vi "GenerateTestAllTask.vi"() -> (3 "Task Out":refnum<k21>)   [LabVIEW 2013]
uses:
  <vilib>/DAQmx/create/channels.llb/DAQmx Create Channel (AI-Voltage-Basic).vi
  <vilib>/DAQmx/create/channels.llb/DAQmx Create Channel (AI-Strain-Strain Gage).vi
  <vilib>/DAQmx/create/channels.llb/DAQmx Create Channel (AI-Position-LVDT).vi
  <vilib>/DAQmx/create/channels.llb/DAQmx Create Channel (AI-Position-RVDT).vi
  Instance           1 27Saved   GenerateTestAllTask .vi
  <resource>/objmgr/daqmx.rc
  Popups/Progress Bar Actions.ctl
  Data Access Objects/Channel Paths/Channel Path List Actions.ctl
panel:
  out "error out":errorcluster
  in  "error in (no error)":errorcluster
  out "Name":string
  out "AI.MeasType":i32(ring)=10300 items=["Voltage"=10322, "Current"=10134, "More:Voltage:Custom with Excitation"=10323, "Frequency"=10181, "Resistance"=10278, "Temperature:Thermocouple"=10303, "Temperature:Thermistor"=10302, "Temperature:RTD"=10301, "Temperature:Built-in Sensor"=10311, "Strain Gage"=10300, "Position:LVDT"=10352, "Position:RVDT"=10353, "Accelerometer"=10356, "Sound Pressure:Microphone"=10354, "TEDS Sensor"=12531]
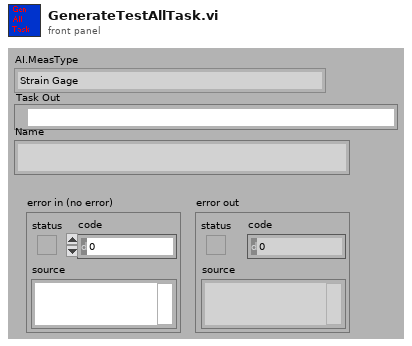
[diagram p1: front panel]
types:
  T1 = typedef "Channel Path List Actions.ctl" = enum16{"Set List", "Get Cont List", "Get Step List", "Get OM List", "Get All List", "Get Exc List", "Get Base List", "Sort List"}
  T2 = typedef "Progress Bar Actions.ctl" = enum16{"Get", "Set", "Exit", "Init"}
  T3 = cluster{"gage factor":dbl, "nominal gage resistance":dbl, "poisson ratio":dbl}
  T4 = cluster{"strain configuration":i32, "lead wire resistance":dbl, "initial bridge voltage":dbl, "voltage excitation source":i32, "voltage excitation value":dbl}
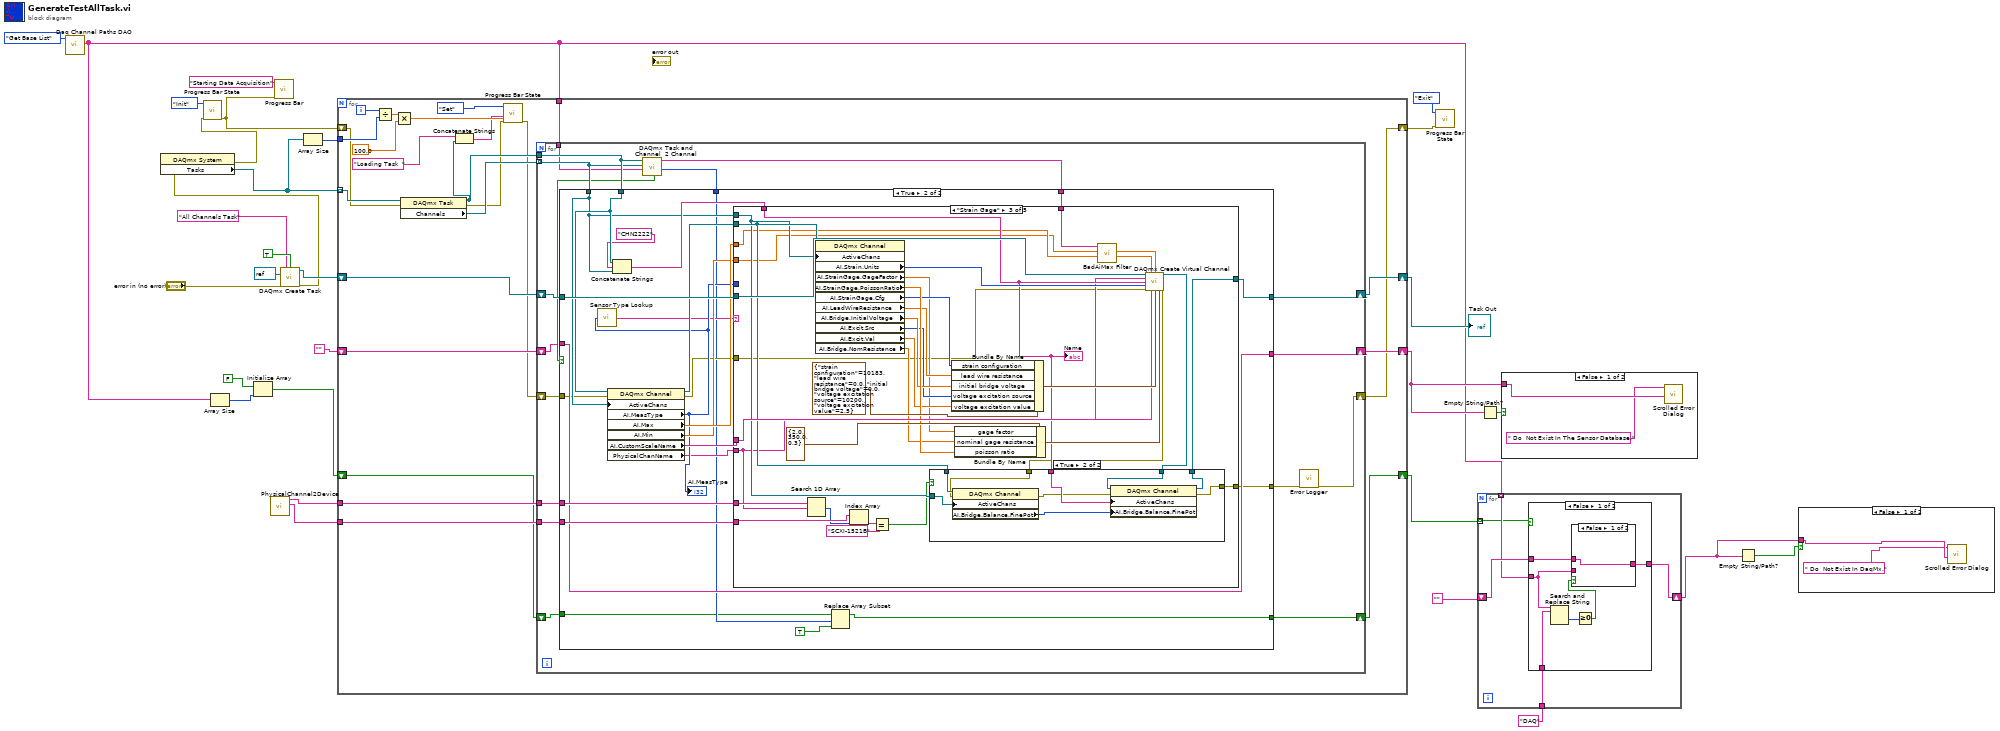
[diagram p0: block diagram]
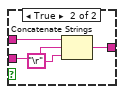
[diagram p3: hidden frame]
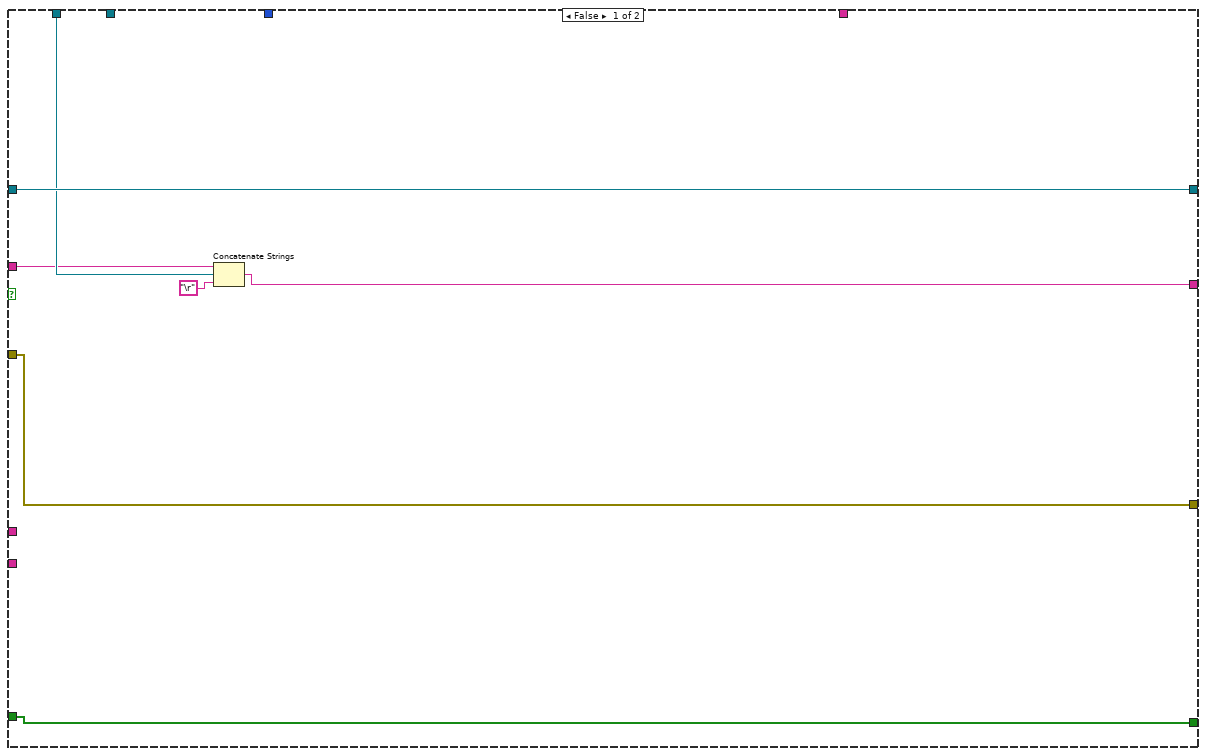
[diagram p6: hidden frame]
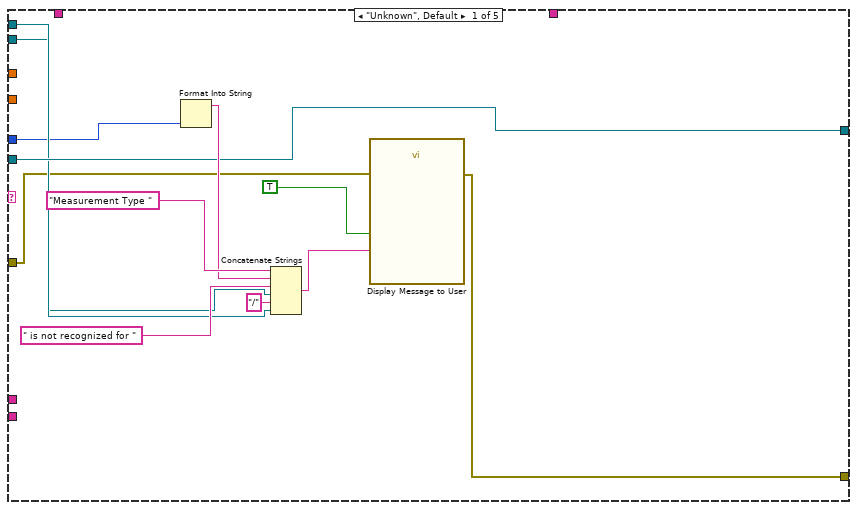
[diagram p7: hidden frame]
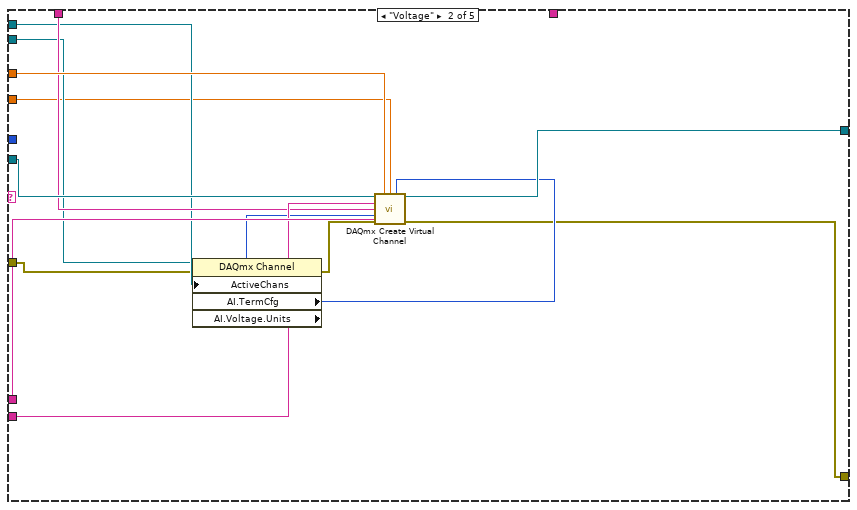
[diagram p8: hidden frame]
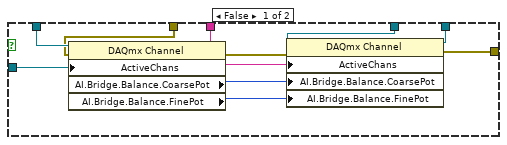
[diagram p9: hidden frame]
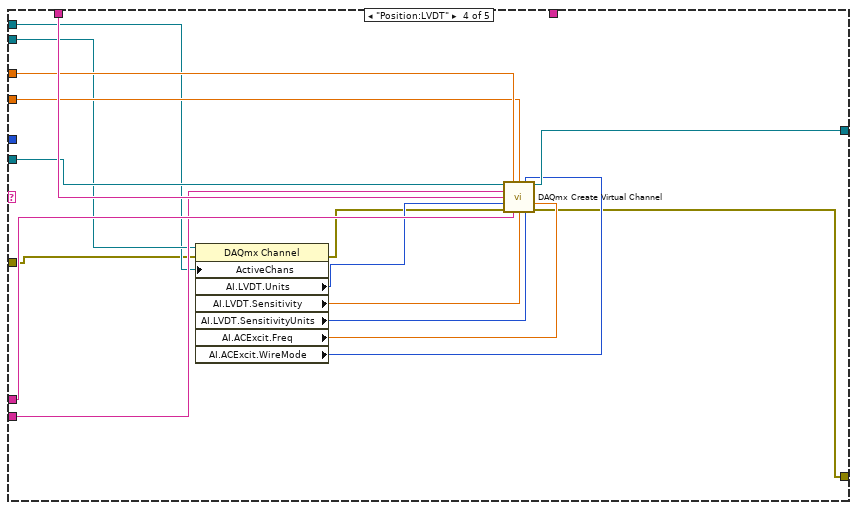
[diagram p10: hidden frame]
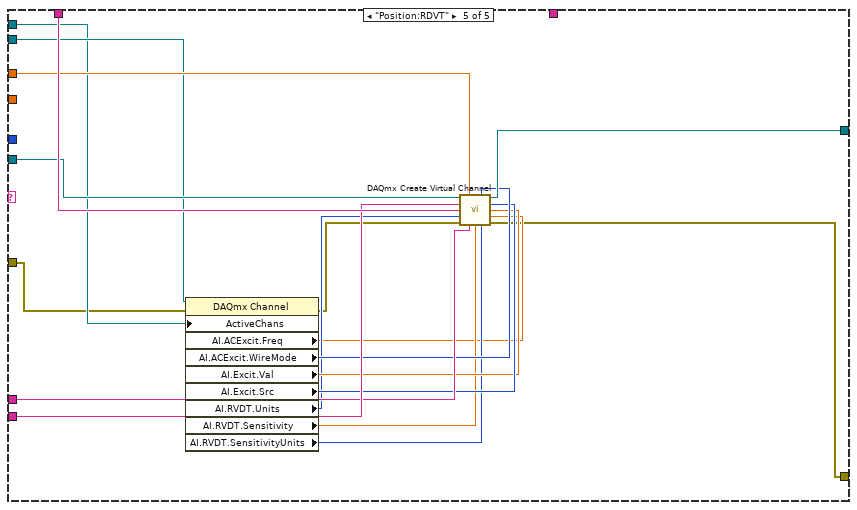
[diagram p11: hidden frame]
diagram:
  n1 = call "Daq Channel Paths DAO.vi"("Actions"=Channel_Path_List_Actions."Get Base List") -> ("Channel Path List Out"=w7:string[])  [unwired: 9 in, 1 out]
  n2 = Array Size(array=w7) -> (size(s)=w10:i32)
  n3 = Initialize Array(FALSE, w10) -> (w8:bool[])
  n4 = call "PhysicalChannel2Device.vi"() -> ("Associated Device"=w24:string[], "Physical Channels"=w25:tag[])  [unwired: 10 out]
  n5 = call <vilib>:"DAQmx Create Task.vi"("new task name"="All Channels Task", "auto cleanup"=TRUE, "task to copy"=refnum<k21> refnum, "error in"="error in (no error)") -> ("task out"=w28:refnum<k21>, "error out"=w12:errorcluster)  [unwired: 1 in, 9 out]
  n6 = property class="DAQmx System"(error in=w12) -> (error out=w11:errorcluster, "Tasks"=w19:refnum<k21>[])  [unwired: 1 in, 1 out]
  n7 = call "Progress Bar State.vi"("error in (no error)"=w11, "Progress Actions"=Progress_Bar_Actions."Init") -> ("error out"=w15:errorcluster)  [unwired: 2 in, 7 out]
  n8 = call "Progress Bar.vi"("error in (no error)"=w15, "Label In"="Starting Data Acquisition") -> ()  [unwired: 10 out]
  n9 = Array Size(array=w19) -> (size(s)=w18:i32)
  n10 = for {
    tunnel: w19 -> [w54] mode=indexing
    shift-right: [w51] -> w27
    shift-left: w28 -> [w52]
    tunnel: w25 -> [w50]
    tunnel: w24 -> [w49]
    shift-right: [w47] -> w22
    shift-left: "" -> [w48]
    tunnel: w18 -> [w44]
    shift-right: [w33] -> w17
    shift-left: w15 -> [w36]
    tunnel: w7 -> [w37]
    shift-right: [w31] -> w6
    shift-left: w8 -> [w32]
    i -> [w45]
    n11 = Divide(x=w45, y=w44) -> (x/y=w43:dbl)
    n12 = Multiply(x=w43, y=100.0) -> (x*y=w41:dbl)
    n13 = property class="DAQmx Task"(reference=w54, error in=w36) -> (reference out=w39:refnum<k21>, error out=w35:errorcluster, "Channels"=w53:refnum<k21>[])
    n14 = Concatenate Strings("Loading Task  " ("string"), w39) -> (w38:string)
    n15 = call "Progress Bar State.vi"("error in (no error)"=w35, "String In"=w38, "Progress In"=w41, "Progress Actions"=Progress_Bar_Actions."Set") -> ("error out"=w34:errorcluster)  [unwired: 7 out]
    n16 = for {
      tunnel: w53 -> [w68] mode=indexing
      tunnel: w39 -> [w69]
      shift-right: [w70] -> w51
      shift-left: w52 -> [w71]
      tunnel: w50 -> [w66]
      tunnel: w49 -> [w65]
      shift-right: [w63] -> w47
      shift-left: w48 -> [w64]
      tunnel: w37 -> [w62]
      shift-right: [w59] -> w33
      shift-left: w34 -> [w61]
      shift-right: [w55] -> w31
      shift-left: w32 -> [w56]
      n17 = call "DAQmx Task and Channel  2 Channel.vi"("Channel Path List In"=w62, "Channel In"=w68, "DAQmx Task Name"=w69) -> ("Channel Name Index"=w57:i32, "Channel Out"=w58:string, "Exists"=w67:bool)  [unwired: 6 out]
      n18 = case shown="True" w67 {
        tunnel: w71 -> [w78 w102]
        tunnel: [w78 w101] -> w70
        tunnel: w69 -> [_ w98]
        tunnel: w68 -> [w77 w95]
        tunnel: w66 -> [_ w89]
        tunnel: w65 -> [_ w88]
        tunnel: w64 -> [w75 w87]
        tunnel: [w74 w87] -> w63
        tunnel: w61 -> [w73 w86]
        tunnel: [w73 w84] -> w60
        tunnel: w58 -> [_ w83]
        tunnel: w57 -> [_ w82]
        tunnel: w56 -> [w72 w81]
        tunnel: [w72 w79] -> w55
        frame False {
          n19 = Concatenate Strings(w75, w77, "\r") -> (w74:string)
        }
        frame True {
          n20 = property class="DAQmx Channel"(reference=w98, error in=w86, "ActiveChans"=w95) -> (reference out=w94:refnum<k21>, error out=w85:errorcluster, "AI.MeasType"=w92:i32, "AI.Max"=w100:dbl, "AI.Min"=w93:dbl, "AI.CustomScaleName"=w99:tag, "PhysicalChanName"=w90:tag)
          "AI.MeasType" <- w92
          n21 = call "Sensor Type Lookup.vi"("AI.MeasType"=w92) -> ("String Rep"=w91:string)
          n22 = Concatenate Strings(w98, "CHN2222", w95) -> (w97:string)
          n23 = case shown="\"Strain Gage\"" w91 {
            tunnel: w102 -> [w109 w128 w163 w190 w215]
            tunnel: [w109 w127 w145 w195 w212] -> w101
            tunnel: w100 -> [_ w126 w130 w198 w216]
            tunnel: w99 -> [_ w125 w158 w197 w213]
            tunnel: w90 -> [_ w124 w141 w196 w214]
            tunnel: w97 -> [_ w123 w146 w199 w217]
            tunnel: w95 -> [w107 w122 w147 w186 w203]
            tunnel: w94 -> [w106 w119 w148 w188 w205]
            tunnel: w93 -> [_ w118 w129 w189 _]
            tunnel: w92 -> [w105 _ _ _ _]
            tunnel: w89 -> [_ _ w143 _ _]
            tunnel: w88 -> [_ _ w142 _ _]
            tunnel: w85 -> [w104 w117 w136 w185 w202]
            tunnel: [w103 w115 w134 w183 w200] -> w84
            tunnel: w83 -> [_ _ w133 _ _]
            frame "Unknown", Default {
              n24 = Format Into String(w105) -> (resulting string=w113:string)  [unwired: 3 in, 1 out]
              n25 = Concatenate Strings("Measurement Type " ("string"), w113, " is not recognized for " ("string"), w106, "/" ("string"), w107) -> (w111:string)
              n26 = call "Display Message to User"("error in (no error)"=w104, "Enable"=TRUE, "Message"=w111) -> ("error out"=w103:errorcluster)  [unwired: 8 out]
            }
            frame "Voltage" {
              n27 = property class="DAQmx Channel"(reference=w119, error in=w117, "ActiveChans"=w122) -> (error out=w116:errorcluster, "AI.TermCfg"=w121:i32, "AI.Voltage.Units"=w120:i32)  [unwired: 1 out]
              n28 = call-poly <vilib>:"DAQmx Create Virtual Channel.vi"("task in"=w128, "maximum value"=w126, "minimum value"=w118, "input terminal configuration"=w121, "physical channels"=w124, "name to assign"=w123, "units"=w120, "error in"=w116, "custom scale name"=w125) -> ("task out"=w127:refnum<k21>, "error out"=w115:errorcluster)  [unwired: 5 out]
            }
            frame "Strain Gage" {
              n29 = Search 1D Array(1D array=w143, element=w141) -> (index of element=w140:i32)  [unwired: 1 out]
              n30 = property class="DAQmx Channel"(reference=w148, "ActiveChans"=w147) -> ("AI.Strain.Units"=w151:i32, "AI.StrainGage.GageFactor"=w150:dbl, "AI.StrainGage.PoissonRatio"=w157:dbl, "AI.StrainGage.Cfg"=w156:i32, "AI.LeadWireResistance"=w155:dbl, "AI.Bridge.InitialVoltage"=w154:dbl, "AI.Excit.Src"=w153:i32, "AI.Excit.Val"=w152:dbl, "AI.Bridge.NomResistance"=w149:dbl)  [unwired: 1 in, 2 out]
              n31 = Index Array(array=w142, index=w140) -> (element=w139:string)
              n32 = Equal?(x=w139, y="SCXI-1521B") -> (x = y?=w137:bool)
              n33 = Bundle By Name(cluster=T4 {"strain configuration"=10183, "lead wire resistance"=0.0, "initial bridge voltage"=0.0, "voltage excitation source"=10200, "voltage excitation value"=2.5} ("bridge information"), "strain configuration"=w156, "lead wire resistance"=w155, "initial bridge voltage"=w154, "voltage excitation source"=w153, "voltage excitation value"=w152) -> (w161:T4)
              n34 = Bundle By Name(cluster=T3 {"gage factor"=2.0, "nominal gage resistance"=350.0, "poisson ratio"=0.3} ("strain gage information"), "gage factor"=w150, "nominal gage resistance"=w149, "poisson ratio"=w157) -> (w159:T3)
              n35 = call "BadAiMax Filter.vi"("Max In"=w130, "Min In"=w129, "Channel Name"=w133) -> ("Max Out"=w131:dbl, "Min Out"=w132:dbl)  [unwired: 6 in, 1 out]
              n36 = call-poly <vilib>:"DAQmx Create Virtual Channel.vi"("task in"=w163, "maximum value"=w131, "minimum value"=w132, "physical channels"=w141, "name to assign"=w146, "units"=w151, "error in"=w136, "custom scale name"=w158, "bridge information"=w161, "strain gage information"=w159) -> ("task out"=w144:refnum<k21>, "error out"=w135:errorcluster)  [unwired: 1 in, 3 out]
              n37 = case shown="True" w137 {
                tunnel: w148 -> [w173 w177]
                tunnel: w147 -> [w172 w178]
                tunnel: w146 -> [w171 w181]
                tunnel: w144 -> [w169 w180]
                tunnel: [w168 w179] -> w145
                tunnel: w135 -> [w166 w176]
                tunnel: [w164 w174] -> w134
                frame False {
                  n38 = property class="DAQmx Channel"(reference=w173, error in=w166, "ActiveChans"=w172) -> (error out=w165:errorcluster, "AI.Bridge.Balance.CoarsePot"=w170:i32, "AI.Bridge.Balance.FinePot"=w167:i32)  [unwired: 1 out]
                  n39 = property class="DAQmx Channel"(reference=w169, error in=w165, "ActiveChans"=w171, "AI.Bridge.Balance.CoarsePot"=w170, "AI.Bridge.Balance.FinePot"=w167) -> (reference out=w168:refnum<k21>, error out=w164:errorcluster)
                }
                frame True {
                  n40 = property class="DAQmx Channel"(reference=w177, error in=w176, "ActiveChans"=w178) -> (error out=w175:errorcluster, "AI.Bridge.Balance.FinePot"=w182:i32)  [unwired: 1 out]
                  n41 = property class="DAQmx Channel"(reference=w180, error in=w175, "ActiveChans"=w181, "AI.Bridge.Balance.FinePot"=w182) -> (reference out=w179:refnum<k21>, error out=w174:errorcluster)
                }
              }
              "Name" <- w146
            }
            frame "Position:LVDT" {
              n42 = property class="DAQmx Channel"(reference=w188, error in=w185, "ActiveChans"=w186) -> (error out=w184:errorcluster, "AI.LVDT.Units"=w187:i32, "AI.LVDT.Sensitivity"=w194:dbl, "AI.LVDT.SensitivityUnits"=w193:i32, "AI.ACExcit.Freq"=w192:dbl, "AI.ACExcit.WireMode"=w191:i32)  [unwired: 1 out]
              n43 = call-poly <vilib>:"DAQmx Create Virtual Channel.vi"("task in"=w190, "maximum value"=w198, "minimum value"=w189, "voltage excitation wire mode"=w191, "physical channels"=w196, "name to assign"=w199, "units"=w187, "voltage excitation frequency"=w192, "error in"=w184, "custom scale name"=w197, "sensitivity"=w194, "sensitivity units"=w193) -> ("task out"=w195:refnum<k21>, "error out"=w183:errorcluster)  [unwired: 2 in]
            }
            frame "Position:RDVT" {
              n44 = property class="DAQmx Channel"(reference=w205, error in=w202, "ActiveChans"=w203) -> (error out=w201:errorcluster, "AI.ACExcit.Freq"=w204:dbl, "AI.ACExcit.WireMode"=w211:i32, "AI.Excit.Val"=w209:dbl, "AI.Excit.Src"=w210:i32, "AI.RVDT.Units"=w208:i32, "AI.RVDT.Sensitivity"=w207:dbl, "AI.RVDT.SensitivityUnits"=w206:i32)  [unwired: 1 out]
              n45 = call-poly <vilib>:"DAQmx Create Virtual Channel.vi"("task in"=w215, "maximum value"=w216, "voltage excitation wire mode"=w211, "physical channels"=w214, "voltage excitation source"=w210, "name to assign"=w217, "voltage excitation value"=w209, "units"=w208, "voltage excitation frequency"=w204, "error in"=w201, "custom scale name"=w213, "sensitivity"=w207, "sensitivity units"=w206) -> ("task out"=w212:refnum<k21>, "error out"=w200:errorcluster)  [unwired: 1 in]
            }
          }
          n46 = Replace Array Subset(array=w81, new element=TRUE ("new element/subarray"), index=w82) -> (w79:bool[])
        }
      }
      n47 = call "Error Logger.vi"("error in (no error)"=w60) -> ("error out"=w59:errorcluster)  [unwired: 10 in]
    }
  }
  "Task Out" <- w27
  n48 = call "Progress Bar State.vi"("error in (no error)"=w17, "Progress Actions"=Progress_Bar_Actions."Exit") -> ()  [unwired: 2 in, 8 out]
  n49 = for {
    tunnel: w7 -> [w220] mode=indexing
    tunnel: w6 -> [w219] mode=indexing
    shift-right: [w221] -> w3
    shift-left: "" -> [w222]
    tunnel: "DAQ" ("search string") -> [w218]
    n50 = case shown="False" w219 {
      tunnel: w220 -> [w226 _]
      tunnel: w222 -> [w228 w234]
      tunnel: [w227 w234] -> w221
      tunnel: w218 -> [w225 _]
      frame False {
        n51 = Search and Replace String(input string=w226, search string=w225) -> (offset past replacement=w224:i32)  [unwired: 6 in, 3 out]
        n52 = Greater Or Equal To 0?(x=w224) -> (x >= 0?=w223:bool)
        n53 = case shown="False" w223 {
          tunnel: w228 -> [w229 w232]
          tunnel: [w229 w231] -> w227
          tunnel: w226 -> [_ w230]
          frame False {
          }
          frame True {
            n54 = Concatenate Strings(w232, w230, "\r") -> (w231:string)
          }
        }
      }
      frame True {
      }
    }
  }
  n55 = Empty String/Path?(string/path=w22) -> (empty?=w23:bool)
  n56 = case shown="False" w23 {
    tunnel: w22 -> [w236 _]
    frame False {
      n57 = call "Scrolled Error Dialog.vi"("Channels"=w236, "Title"=" Do  Not Exist In The Sensor Database." ("string")) -> ()  [unwired: 9 in, 1 out]
    }
    frame True {
    }
  }
  n58 = Empty String/Path?(string/path=w3) -> (empty?=w4:bool)
  n59 = case shown="False" w4 {
    tunnel: w3 -> [w238 _]
    frame False {
      n60 = call "Scrolled Error Dialog.vi"("Channels"=w238, "Title"=" Do  Not Exist In DaqMx." ("string")) -> ()  [unwired: 9 in, 1 out]
    }
    frame True {
    }
  }
